vi "Set Request ID.vi"(8 "error in (no error)":errorcluster, 10 "Request ID":string, 11 "Request in":refnum<class "Request.lvclass">) -> (0 "error out":errorcluster, 3 "Request out":refnum<class "Request.lvclass">)   [LabVIEW 2020, in "obs-websocket.lvlib" / "Request.lvclass"]
uses:
  Request.lvclass
  Request.lvclass/Request.ctl
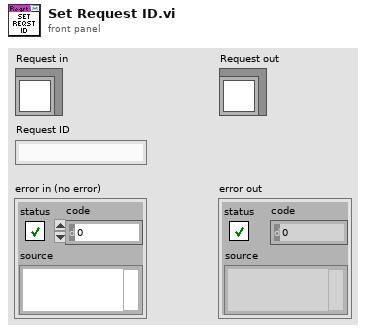
[diagram p1: front panel]
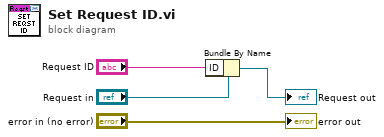
[diagram p0: block diagram]
diagram:
  n1 = Bundle By Name(cluster="Request in", "ID"="Request ID") -> (→"Request out":refnum<class "Request.lvclass">)
  "error out" <- "error in (no error)"
